vi "AdjustPS-better.vi"(1 "Number of steps":dbl=3.0, 2 "Power Supply Address":string="6", 3 "Gaussmeter Address":string="22", 4 "Field Set Point (Oe)":dbl) -> (0 "Set PS to (A)":dbl)   [LabVIEW 2015]
panel:
  out "Current PS Output (A)":dbl
  out "Measured Field (Oe)":dbl
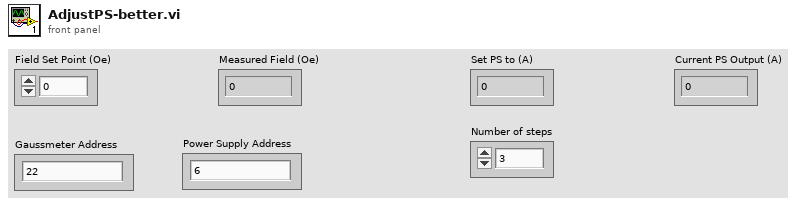
[diagram p1: front panel]
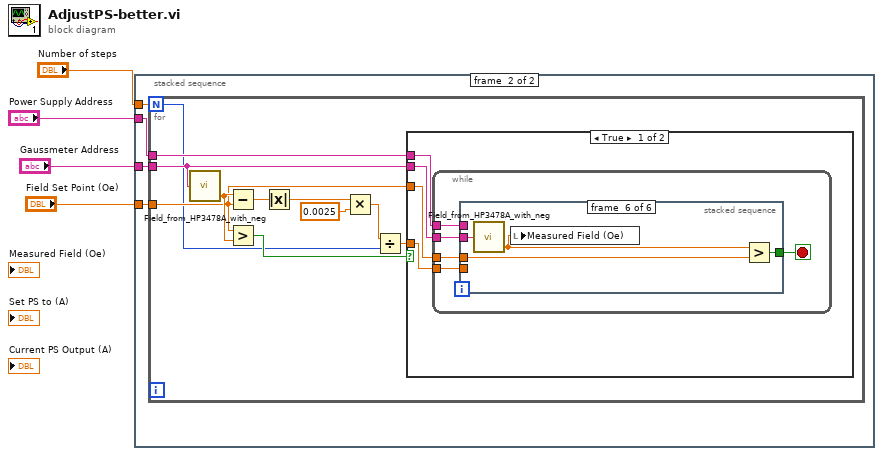
[diagram p0: block diagram]
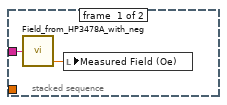
[diagram p2: hidden frame]
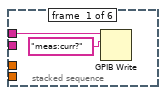
[diagram p3: hidden frame]
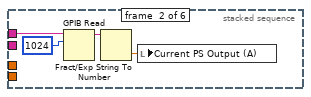
[diagram p4: hidden frame]
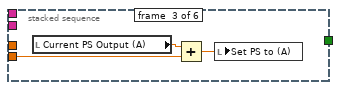
[diagram p5: hidden frame]
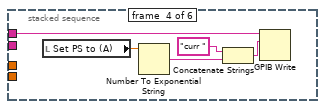
[diagram p6: hidden frame]
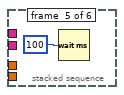
[diagram p7: hidden frame]
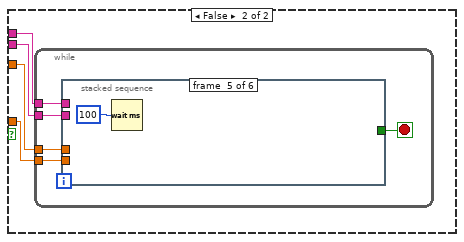
[diagram p8: hidden frame]
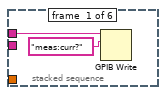
[diagram p9: hidden frame]
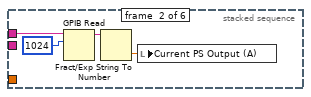
[diagram p10: hidden frame]
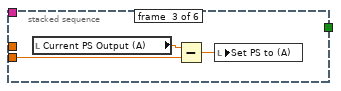
[diagram p11: hidden frame]
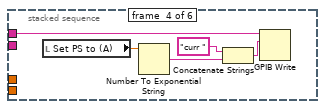
[diagram p12: hidden frame]
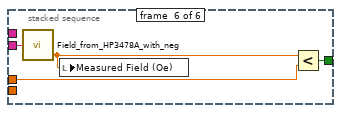
[diagram p13: hidden frame]
diagram:
  n1 = stacked-sequence {
    tunnel: "Gaussmeter Address" -> [w6 w7]
    tunnel: "Field Set Point (Oe)" -> [_ w10]
    tunnel: "Power Supply Address" -> [_ w9]
    tunnel: "Number of steps" -> [_ w8]
    frame #0 {
      n2 = call "Field_from_HP3478A_with_neg.vi"("GPIB Address"=w6) -> ("Oe"=w5:dbl)  [unwired: 2 out]
      n3 = local write "Measured Field (Oe)"(w5) -> ()
    }
    frame #1 {
      n4 = for {
        N: w8 -> [w11]
        tunnel: w7 -> [w19]
        tunnel: w10 -> [w17]
        tunnel: w9 -> [w20]
        n5 = call "Field_from_HP3478A_with_neg.vi"("GPIB Address"=w19) -> ("Oe"=w18:dbl)  [unwired: 2 out]
        n6 = Subtract(x=w18, y=w17) -> (x-y=w16:dbl)
        n7 = Greater?(x=w17, y=w18) -> (0:w21:bool)
        n8 = Absolute Value(x=w16) -> (abs(x)=w15:dbl)
        n9 = Multiply(x=w15, y=0.0025) -> (x*y=w13:dbl)
        n10 = Divide(x=w13, y=w11) -> (x/y=w12:dbl)
        n11 = case shown="True" w21 {
          tunnel: w20 -> [w25 w53]
          tunnel: w12 -> [w24 w52]
          tunnel: w19 -> [w23 w51]
          tunnel: w17 -> [w22 w50]
          frame True {
            n12 = while {
              tunnel: w25 -> [w30]
              tunnel: w24 -> [w29]
              tunnel: w23 -> [w28]
              tunnel: w22 -> [w27]
              stop <- w26 stop-if-true
              n13 = stacked-sequence {
                tunnel: w30 -> [w31 w34 _ w40 _ _]
                tunnel: w29 -> [_ _ w39 _ _ _]
                tunnel: w28 -> [_ _ _ _ _ w49]
                tunnel: w27 -> [_ _ _ _ _ w47]
                tunnel: [_ _ _ _ _ w46] -> w26
                frame #0 {
                  n14 = GPIB Write(0:w31, 1:"meas:curr?" ("data")) -> ()  [unwired: 3 in, 2 out]
                }
                frame #1 {
                  n15 = GPIB Read(0:w34, 1:1024 ("byte count")) -> (5:w35:string)  [unwired: 3 in, 2 out]
                  n16 = Fract/Exp String To Number(string=w35) -> (number=w33:dbl)  [unwired: 3 in, 1 out]
                  n17 = local write "Current PS Output (A)"(w33) -> ()
                }
                frame #2 {
                  n18 = local read "Current PS Output (A)"() -> (w38:dbl)
                  n19 = Add(x=w38, y=w39) -> (x+y=w37:dbl)
                  n20 = local write "Set PS to (A)"(w37) -> ()
                }
                frame #3 {
                  n21 = local read "Set PS to (A)"() -> (w41:dbl)
                  n22 = Number To Exponential String(number=w41) -> (E-format string=w44:string)  [unwired: 3 in]
                  n23 = Concatenate Strings("curr " ("string"), w44) -> (w42:string)
                  n24 = GPIB Write(0:w40, 1:w42) -> ()  [unwired: 3 in, 2 out]
                }
                frame #4 {
                  n25 = Wait (ms)(milliseconds to wait=u32 100) -> ()  [unwired: 1 out]
                }
                frame #5 {
                  n26 = call "Field_from_HP3478A_with_neg.vi"("GPIB Address"=w49) -> ("Oe"=w48:dbl)  [unwired: 2 out]
                  n27 = local write "Measured Field (Oe)"(w48) -> ()
                  n28 = Greater?(x=w48, y=w47) -> (0:w46:bool)
                }
              }
            }
          }
          frame False {
            n29 = while {
              tunnel: w53 -> [w58]
              tunnel: w52 -> [w57]
              tunnel: w51 -> [w56]
              tunnel: w50 -> [w55]
              stop <- w54 stop-if-true
              n30 = stacked-sequence {
                tunnel: w58 -> [w59 w62 _ w68 _ _]
                tunnel: w57 -> [_ _ w67 _ _ _]
                tunnel: w56 -> [_ _ _ _ _ w77]
                tunnel: w55 -> [_ _ _ _ _ w75]
                tunnel: [_ _ _ _ _ w74] -> w54
                frame #0 {
                  n31 = GPIB Write(0:w59, 1:"meas:curr?" ("data")) -> ()  [unwired: 3 in, 2 out]
                }
                frame #1 {
                  n32 = GPIB Read(0:w62, 1:1024 ("byte count")) -> (5:w63:string)  [unwired: 3 in, 2 out]
                  n33 = Fract/Exp String To Number(string=w63) -> (number=w61:dbl)  [unwired: 3 in, 1 out]
                  n34 = local write "Current PS Output (A)"(w61) -> ()
                }
                frame #2 {
                  n35 = local read "Current PS Output (A)"() -> (w66:dbl)
                  n36 = Subtract(x=w66, y=w67) -> (x-y=w65:dbl)
                  n37 = local write "Set PS to (A)"(w65) -> ()
                }
                frame #3 {
                  n38 = local read "Set PS to (A)"() -> (w69:dbl)
                  n39 = Number To Exponential String(number=w69) -> (E-format string=w72:string)  [unwired: 3 in]
                  n40 = Concatenate Strings("curr " ("string"), w72) -> (w70:string)
                  n41 = GPIB Write(0:w68, 1:w70) -> ()  [unwired: 3 in, 2 out]
                }
                frame #4 {
                  n42 = Wait (ms)(milliseconds to wait=u32 100) -> ()  [unwired: 1 out]
                }
                frame #5 {
                  n43 = call "Field_from_HP3478A_with_neg.vi"("GPIB Address"=w77) -> ("Oe"=w76:dbl)  [unwired: 2 out]
                  n44 = local write "Measured Field (Oe)"(w76) -> ()
                  n45 = Less?(x=w76, y=w75) -> (x < y?=w74:bool)
                }
              }
            }
          }
        }
      }
    }
  }
